vi "Convert State for Save.vi"(2 "Container State":T1 caption="容器状态", 3 "Display State":T2={"method"=enum."None", "current color"=1, "available black position"=[], "available white position"=[], "Interactive Action"=refnum, "row"=0, "column"=0} caption="显示状态") -> (1 "Display State To Save":variant caption="待保存显示状态")   [LabVIEW 2011, in "Othello.xctl"]
uses:
  Othello.xctl
  State.ctl
  Control/Method Call.ctl
  Control/Pict Ring Chess.ctl
  Control/Interactive Action.ctl
  <vilib>/_xctls/Container State.ctl
  <vilib>/_xctls/XControlSupport.lvlib
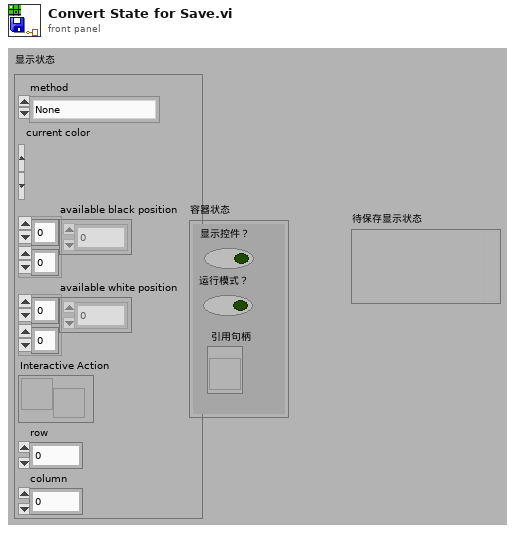
[diagram p1: front panel]
types:
  T1 = typedef "XControlSupport.lvlib/Container State.ctl" = cluster{"Indicator?":bool, "Run Mode?":bool, " Refnum":refnum<vi>}
  T2 = typedef "Othello.xctl/State.ctl" = cluster{"method":T3, "current color":T4, "available black position":i32[][], "available white position":i32[][], "Interactive Action":T5, "row":i32, "column":i32}
  T3 = typedef "Othello.xctl/Method Call.ctl" = enum16{"None", "New Game", "Play One"}
  T4 = typedef "Othello.xctl/Pict Ring Chess.ctl" = u16
  T5 = typedef "Othello.xctl/Interactive Action.ctl" = refnum<user-event>
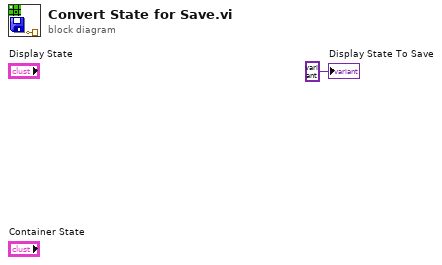
[diagram p0: block diagram]
diagram:
  "Display State To Save" <- variant ("Display State To Save")
